vi "Apply Leverage Force.vi"(10 "force":dbl, 11 "Pryable in":refnum<class "Pryable.lvclass">) -> (3 "Pryable out":refnum<class "Pryable.lvclass">)   [LabVIEW 2023, in "Pryable.lvclass"]
uses:
  Pryable.lvclass
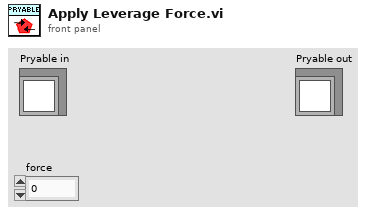
[diagram p1: front panel]
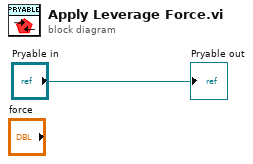
[diagram p0: block diagram]
diagram:
  "Pryable out" <- "Pryable in"
